vi "Config Measure Harmonics.vi"(0 "VISA resource name":refnum<visa-resource-name>, 1 "Min Order (0)":u16 max=1, 2 "Max Order (1)":i16=1 min=1 max=500 step=1, 11 "error in (no error)":errorcluster, 12 "THD (0: Total)":u16(ring) items=["Total", "Fundamental"]) -> (4 "VISA resource name out":refnum<visa-resource-name>, 15 "error out":errorcluster)   [LabVIEW 2013, in "Yokogawa.lvlib" / "Yokogawa PZ4000.lvlib"]
doc: "This VI sends the Measure Harmonics group command to the PZ4000 series."
uses:
  Yokogawa PZ4000.lvlib
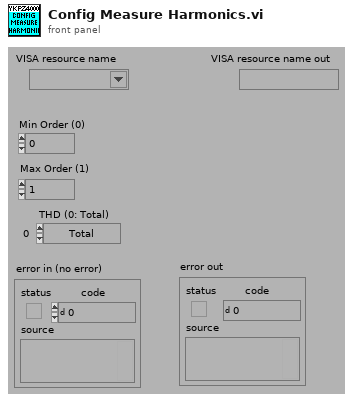
[diagram p1: front panel]
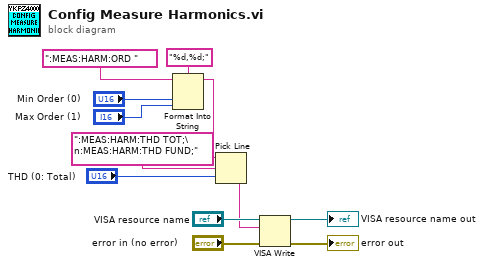
[diagram p0: block diagram]
diagram:
  n1 = Format Into String(format string="%d,%d;", initial string=":MEAS:HARM:ORD ", "Min Order (0)", "Max Order (1)") -> (resulting string=w1:string)  [unwired: 1 in, 1 out]
  n2 = Pick Line(string ("")=w1, multi-line string=":MEAS:HARM:THD TOT;\n:MEAS:HARM:THD FUND;", line index="THD (0: Total)") -> (output string=w2:string)
  n3 = VISA Write(VISA resource name="VISA resource name", write buffer=w2, error in (no error)="error in (no error)") -> (VISA resource name out=→"VISA resource name out":refnum<visa-resource-name>, error out=→"error out":errorcluster)  [unwired: 1 out]
